vi "Get Remote Info.vi"(8 "error in":errorcluster, 11 "NetStream in":refnum<class "NetStream.lvclass">) -> (0 "error out":errorcluster, 1 "Remote Port":u16, 2 "Remote Address":string, 3 "NetStream out":refnum<class "NetStream.lvclass">)   [LabVIEW 2022 SP3, in "hse-network.lvlib" / "NetStream.lvclass"]
doc: "____\nHAMPEL SOFTWARE ENGINEERING v3.8.0 (2023-12-18 14:41)"
uses:
  NetStream.lvclass
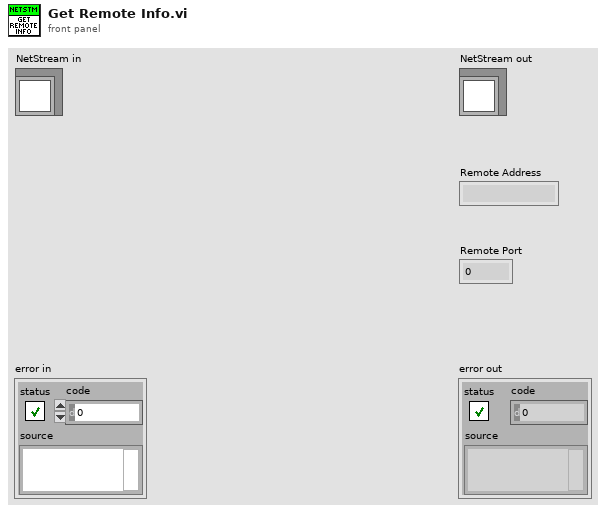
[diagram p1: front panel]
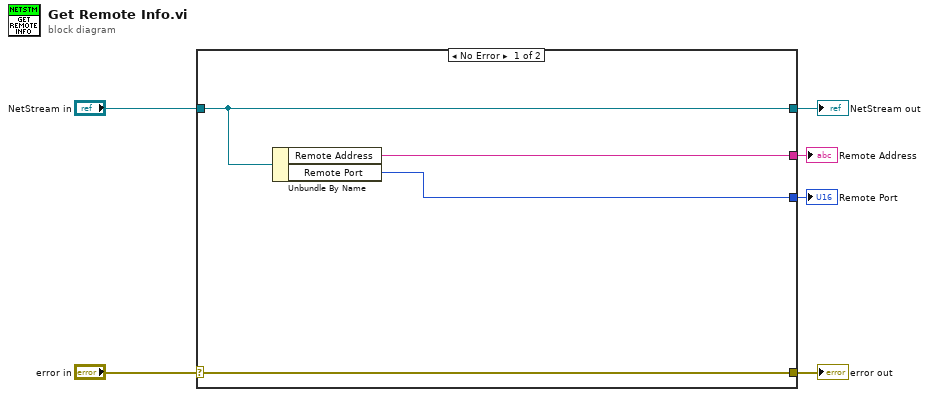
[diagram p0: block diagram]
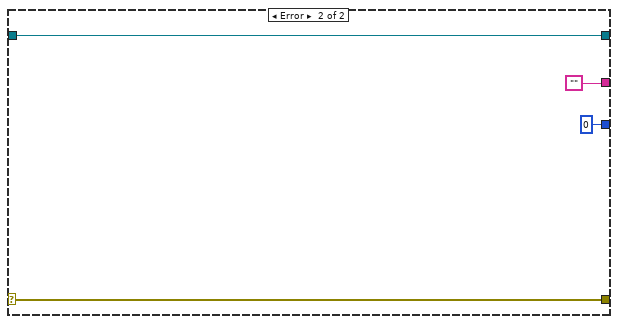
[diagram p2: hidden frame]
diagram:
  n1 = case shown="No Error" "error in" {
    selector: "error in" -> [w10 w14]
    tunnel: [w10 w14] -> w5
    tunnel: [w9 w13] -> w3
    tunnel: "NetStream in" -> [w9 w13]
    tunnel: [w8 ""] -> w2
    tunnel: [w7 u16 0 ("Remote Port")] -> w1
    frame No Error {
      n2 = Unbundle By Name(w9) -> ("Remote Address"=w8:string, "Remote Port"=w7:u16)
    }
    frame Error {
    }
  }
  "error out" <- w5
  "NetStream out" <- w3
  "Remote Address" <- w2
  "Remote Port" <- w1
